vi "Regex verify status.vi"(8 "Error In":errorcluster, 11 "Input String":string) -> (0 "Error Out":errorcluster, 1 "Setpoint/Rate":dbl format="%.5g", 2 "Current":dbl format="%.5g", 3 "Valid Data":bool, 4 "Status":T1)   [LabVIEW 2019]
uses:
  <vilib>/regexp/Match Regular Expression.xnode
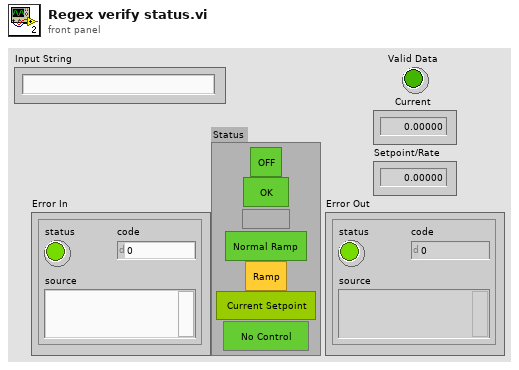
[diagram p1: front panel]
types:
  T1 = cluster{bool, bool, "Ramp Status":u16, bool, bool, bool, bool}
  T2 = cluster{"Boolean array[0]":bool, "Boolean array[1]":bool, "Boolean array[2]":bool, "Boolean array[3]":bool, "Boolean array[4]":bool, "Boolean array[5]":bool, "Boolean array[6]":bool, "Boolean array[7]":bool}
  T3 = cluster{"Boolean array[0]":bool, "Boolean array[1]":bool, u16, "Boolean array[4]":bool, "Boolean array[5]":bool, "Boolean array[6]":bool, "Boolean array[7]":bool}
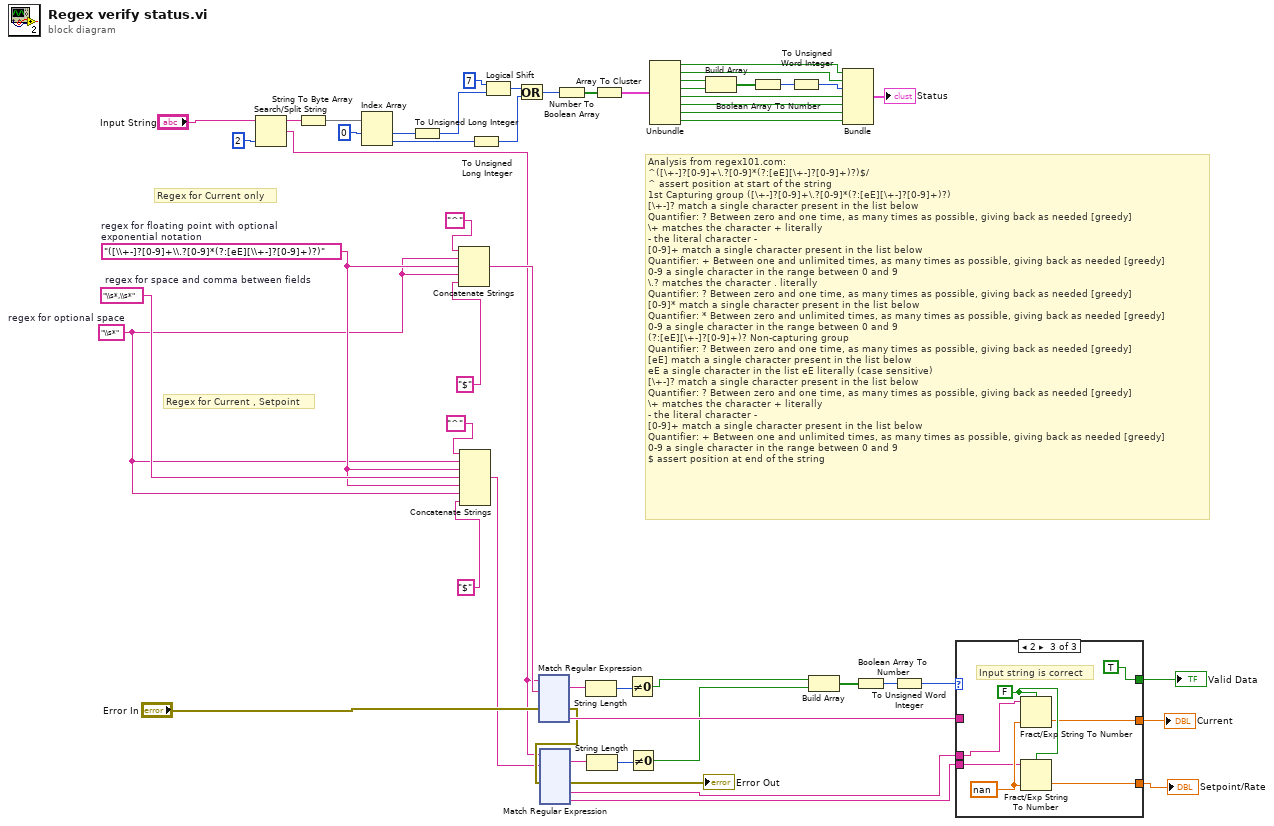
[diagram p0: block diagram]
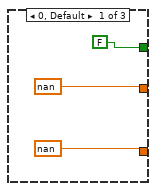
[diagram p2: hidden frame]
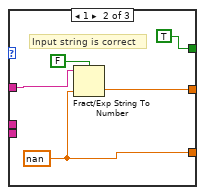
[diagram p3: hidden frame]
diagram:
  w15 = "\\s*"  # regex for optional space
  w17 = "\\s*,\\s*"  # regex for space and comma between fields
  w16 = "([\\+-]?[0-9]+\\.?[0-9]*(?:[eE][\\+-]?[0-9]+)?)"  # regex for floating point with optional exponential notation
  # "Regex for Current , Setpoint"
  # "Regex for Current only"
  # "Analysis from regex101.com:\n^([\\+-]?[0-9]+\\.?[0-9]*(?:[eE][\\+-]?[0-9]+)?)$/\n^ assert position at start of the string\n1st Capturing group ([\\+-]?[0-9]+\\.?[0-9]*(?:[eE][\\+-]?[0-9]+)?)\n[\\+-]? match a single character present in the list below\nQuantifier: ? Between zero and one time, as many times as possible, giving back as needed [greedy]\n\\+ matches the character + literally\n- the literal character -\n[0-9]+ match a single character present in the list below\nQuantifier: + Between one and unlimited times, as many times as possible, giving back as needed [greedy]\n0-9 a single character in the range between 0 and 9\n\\.? matches the character . literally\nQuantifier: ? Between zero and one time, as many times as possible, giving back as needed [greedy]\n[0-9]* match a single character present in the list below\nQuantifier: * Between zero and unlimited times, as many times as possible, giving back as needed [greedy]\n0-9 a single character in the range between 0 and 9\n(?:[eE][\\+-]?[0-9]+)? Non-capturing group\nQuantifier: ? Between zero and one time, as many times as possible, giving back as needed [greedy]\n[eE] match a single character present in the list below\neE a single character in the list eE literally (case sensitive)\n[\\+-]? match a single character present in the list below\nQuantifier: ? Between zero and one time, as many times as possible, giving back as needed [greedy]\n\\+ matches the character + literally\n- the literal character -\n[0-9]+ match a single character present in the list below\nQuantifier: + Between one and unlimited times, as many times as possible, giving back as needed [greedy]\n0-9 a single character in the range between 0 and 9\n$ assert position at end of the string"
  n1 = Search/Split String(string="Input String", offset (0)=2) -> (substring before match=w46:string, match + rest of string=w2:string)  [unwired: 1 in, 1 out]
  n2 = String To Byte Array(string=w46) -> (unsigned byte array=w42:u8[])
  n3 = Index Array(array=w42, index #1=0) -> (element #1=w41:u8, element #2=w23:u8)  [unwired: 1 in]
  n4 = To Unsigned Long Integer(number=w41) -> (unsigned 32bit integer=w24:u32)
  n5 = Concatenate Strings("^", w15, w16, w15, "$") -> (w54:string)
  n6 = Concatenate Strings("^", w15, w16, w17, w16, w15, "$") -> (w1:string)
  n7 = To Unsigned Long Integer(number=w23) -> (unsigned 32bit integer=w25:u32)
  n8 = Logical Shift(y=u8 7, x=w24) -> (x << y=w39:u32)
  n9 = Or(x=w39, y=w25) -> (x .or. y?=w44:u32)
  n10 = xnode "Match Regular Expression"("input string"=w2, "regular expression"=w54, "error in"="Error In") -> ("whole match"=w51:string, "error out"=w11:errorcluster, "submatch 1"=w52:string)  [unwired: 3 in, 3 out]
  n11 = xnode "Match Regular Expression"("input string"=w2, "regular expression"=w1, "error in"=w11) -> ("whole match"=w13:string, "error out"=→"Error Out":errorcluster, "submatch 1"=w3:string, "submatch 2"=w4:string)  [unwired: 3 in, 3 out]
  n12 = Number To Boolean Array(number=w44) -> (Boolean array=w45:bool[])
  n13 = String Length(string=w51) -> (length=w50:i32)
  n14 = String Length(string=w13) -> (length=w12:i32)
  n15 = Array To Cluster(array=w45) -> (cluster=w37:T2)
  n16 = Not Equal To 0?(x=w50) -> (x != 0?=w7:bool)
  n17 = Not Equal To 0?(x=w12) -> (x != 0?=w6:bool)
  n18 = Unbundle(w37) -> ("Boolean array[0]"=w32:bool, "Boolean array[1]"=w31:bool, "Boolean array[2]"=w34:bool, "Boolean array[3]"=w33:bool, "Boolean array[4]"=w29:bool, "Boolean array[5]"=w28:bool, "Boolean array[6]"=w27:bool, "Boolean array[7]"=w26:bool)
  n19 = Build Array(w34, w33) -> (w35:bool[])
  n20 = Boolean Array To Number(Boolean array=w35) -> (number=w36:u32)
  n21 = To Unsigned Word Integer(number=w36) -> (unsigned 16bit integer=w30:u16)
  n22 = Build Array(w7, w6) -> (w8:bool[])
  n23 = Bundle("Boolean array[0]"=w32, "Boolean array[1]"=w31, w30, "Boolean array[4]"=w29, "Boolean array[5]"=w28, "Boolean array[6]"=w27, "Boolean array[7]"=w26) -> (→"Status":T3)  [unwired: 1 in]
  n24 = Boolean Array To Number(Boolean array=w8) -> (number=w9:u32)
  n25 = To Unsigned Word Integer(number=w9) -> (unsigned 16bit integer=w5:u16)
  n26 = case shown="2" w5 {
    tunnel: w52 -> [_ w61 _]
    tunnel: w4 -> [_ _ w67]
    tunnel: [FALSE TRUE TRUE] -> w48
    tunnel: [nan ("Setpoint") w58 w65] -> w20
    tunnel: [nan ("Setpoint") w59 w64] -> w21
    tunnel: w3 -> [_ _ w63]
    frame 0, Default {
    }
    frame 1 {
      w58 = nan ("Setpoint")
      # "Input string is correct"
      n27 = Fract/Exp String To Number(use system decimal point (T)=FALSE, string=w61, default (0 dbl)=w58) -> (number=w59:dbl)  [unwired: 1 in, 1 out]
    }
    frame 2 {
      w68 = nan ("Setpoint")
      w66 = FALSE ("use system decimal point (T)")
      # "Input string is correct"
      n28 = Fract/Exp String To Number(use system decimal point (T)=w66, string=w63, default (0 dbl)=w68) -> (number=w64:dbl)  [unwired: 1 in, 1 out]
      n29 = Fract/Exp String To Number(use system decimal point (T)=w66, string=w67, default (0 dbl)=w68) -> (number=w65:dbl)  [unwired: 1 in, 1 out]
    }
  }
  "Valid Data" <- w48
  "Current" <- w21
  "Setpoint/Rate" <- w20
